vi "PV ModulLine Data.vi"(8 "error in (no error)":errorcluster, 9 "PV ModulLine-Cluster":T1={"Parameter"=enum." Pressure  [mbar] (740)", "Parameter\nread only<->describe"=FALSE, "Correction facktor\n(0,20 - 9,90) "=1.0} {"Correction facktor\n(0,20 - 9,90)" min=0.2 max=9.9 step=0.01 format="%.2f"}, 10 "Adress of unit":u16=10 max=999 step=1, 11 "VISA session":refnum<visa-resource-name>) -> (0 "error out":errorcluster, 2 "response (data)":string, 3 "dup VISA session":refnum<visa-resource-name>)   [LabVIEW 2021, in "Pfeiffer Vacuum.lvlib"]
doc: "There are 5 parameters available, only one of which can be enabled at a time. \n\n0 - Pressure [mbar] (default) (740)\n1 - Correction factor sensor 1..6 (742)\n2 - Actual error code (read only) (303)\n3 - Software version Transmitter (read only) (312)\n4 - Unit type Transmitter (read only) (349)\n\nNote: The controls right of this one will set the appropriate values for the selected parameter. Any settings for an parameter that is not selected will be ignored. If a value is out of range, it will be changed to either the upper or the lower limit of the range."
uses:
  <instrlib>/Pfeiffer Vacuum/Pfeiffer Vacuum.lvlib
  <instrlib>/Pfeiffer Vacuum/Public/ModulLine/PV ModulLine - Cluster.ctl
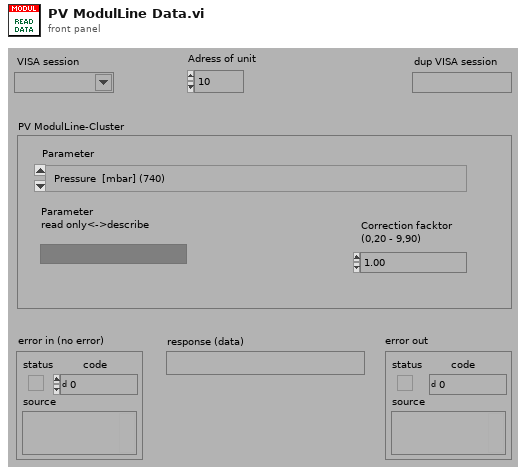
[diagram p1: front panel]
types:
  T1 = typedef "Pfeiffer Vacuum.lvlib/PV ModulLine - Cluster.ctl" = cluster{"Parameter":enum16{" Pressure  [mbar] (740)", " Correction factor sensor (742)", " Actual error code (read only) (303)", " Software version Transmitter (read only) (312)", " Unit type Transmitter (read only) (349)"}, "Parameter\nread only<->describe":bool, "Correction facktor\n(0,20 - 9,90) ":sgl}
  T2 = enum16{" Pressure  [mbar] (740)", " Correction factor sensor (742)", " Actual error code (read only) (303)", " Software version Transmitter (read only) (312)", " Unit type Transmitter (read only) (349)"}
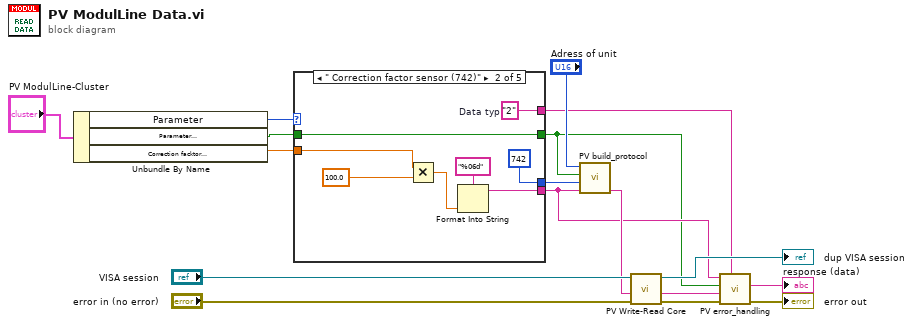
[diagram p0: block diagram]
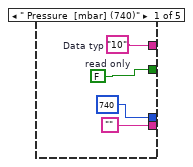
[diagram p2: hidden frame]
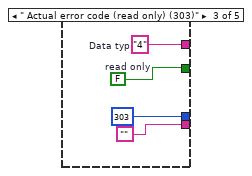
[diagram p3: hidden frame]
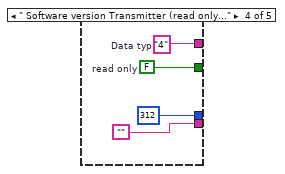
[diagram p4: hidden frame]
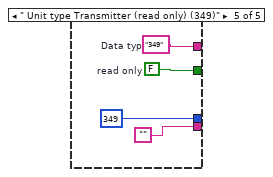
[diagram p5: hidden frame]
diagram:
  n1 = Unbundle By Name("PV ModulLine-Cluster") -> ("Parameter"=w15:T2, "Parameter\nread only<->describe"=w14:bool, "Correction facktor\n(0,20 - 9,90)"=w2:sgl)
  n2 = case shown="\" Correction factor sensor (742)\"" w15 {
    tunnel: [u16 740 ("Parameter-number") u16 742 ("Parameter-number") u16 303 ("Parameter-number") u16 312 ("Parameter-number") u16 349 ("Parameter-number")] -> w16
    tunnel: ["" w22 "" "" ""] -> w5
    tunnel: [w18 w28 w32 w35 w41] -> w4
    tunnel: w14 -> [_ w28 _ _ _]
    tunnel: w2 -> [_ w24 _ _ _]
    tunnel: [w20 w27 w30 w34 w38] -> w6
    frame " Pressure  [mbar] (740)" {
      w18 = FALSE  # read only
      w20 = "10"  # Data typ
    }
    frame " Correction factor sensor (742)" {
      w27 = "2"  # Data typ
      n3 = Multiply(x=w24, y=100.0) -> (x*y=w23:dbl)
      n4 = Format Into String(format string="%06d" ("Format-String"), w23) -> (resulting string=w22:string)  [unwired: 2 in, 1 out]
    }
    frame " Actual error code (read only) (303)" {
      w30 = "4"  # Data typ
      w32 = FALSE  # read only
    }
    frame " Software version Transmitter (read only) (312)" {
      w34 = "4"  # Data typ
      w35 = FALSE  # read only
    }
    frame " Unit type Transmitter (read only) (349)" {
      w38 = "349"  # Data typ
      w41 = FALSE  # read only
    }
  }
  n5 = call <instrlib>:"PV build_protocol.vi"("Data"=w5, "Parameter-number"=w16, "parameter\nread<->describe"=w4, "Adress"="Adress of unit") -> ("output"=w10:string)  [unwired: 3 in]
  n6 = call <instrlib>:"PV Write-Read Core.vi"("error in"="error in (no error)", "Write data in"=w10, "VISA session"="VISA session") -> ("error out"=w7:errorcluster, "response (data) out"=w8:string, "dup VISA session"=→"dup VISA session":refnum<visa-resource-name>)  [unwired: 2 in]
  n7 = call <instrlib>:"PV error_handling.vi"("Data Typ in"=w6, "error in"=w7, "response (data) in"=w8, "Parameter\nread only<->describe"=w4, "data in"=w5) -> ("error out"=→"error out":errorcluster, "Data out"=→"response (data)":string)  [unwired: 4 in, 1 out]
